vi "Read XML HW Configuration File.vi"(8 "error in (no error)":errorcluster, 10 "XML Configuration File Path":path=path "D:/1553 CD/HW Reference files/1553_HW_Reference_001.xml") -> (0 "error out":errorcluster, 3 "channels":T1[](array[typedef]))   [LabVIEW 2020, in "Ballard 1553 System Explorer.lvlib"]
uses:
  Ballard 1553 System Explorer.lvlib
  Ballard_Channel.ctl
  Ballard_BC.ctl
  Ballard_message.ctl
  Ballard_messageType.ctl
  Ballard_CWD1.ctl
  Ballard_CWD2.ctl
  Ballard_minorFrame.ctl
  Ballard_majorFrame.ctl
  Ballard_acyclicFrame.ctl
  Ballard_RT.ctl
  Ballard_RT subAddress.ctl
  Ballard_RT direction.ctl
  Ballard_RT rtMode.ctl
  Ballard_RT modeCode.ctl
  C:/Users/Administrator/Desktop/GIT/Ballard-MIL-STD-1553-Custom-Device/Source/System Explorer/SubVIs/Parse XML Ballard/1.2/BTIXML_SerDes.dll
  1.2/BTIXML_SerDes.dll
panel:
  out "name":string
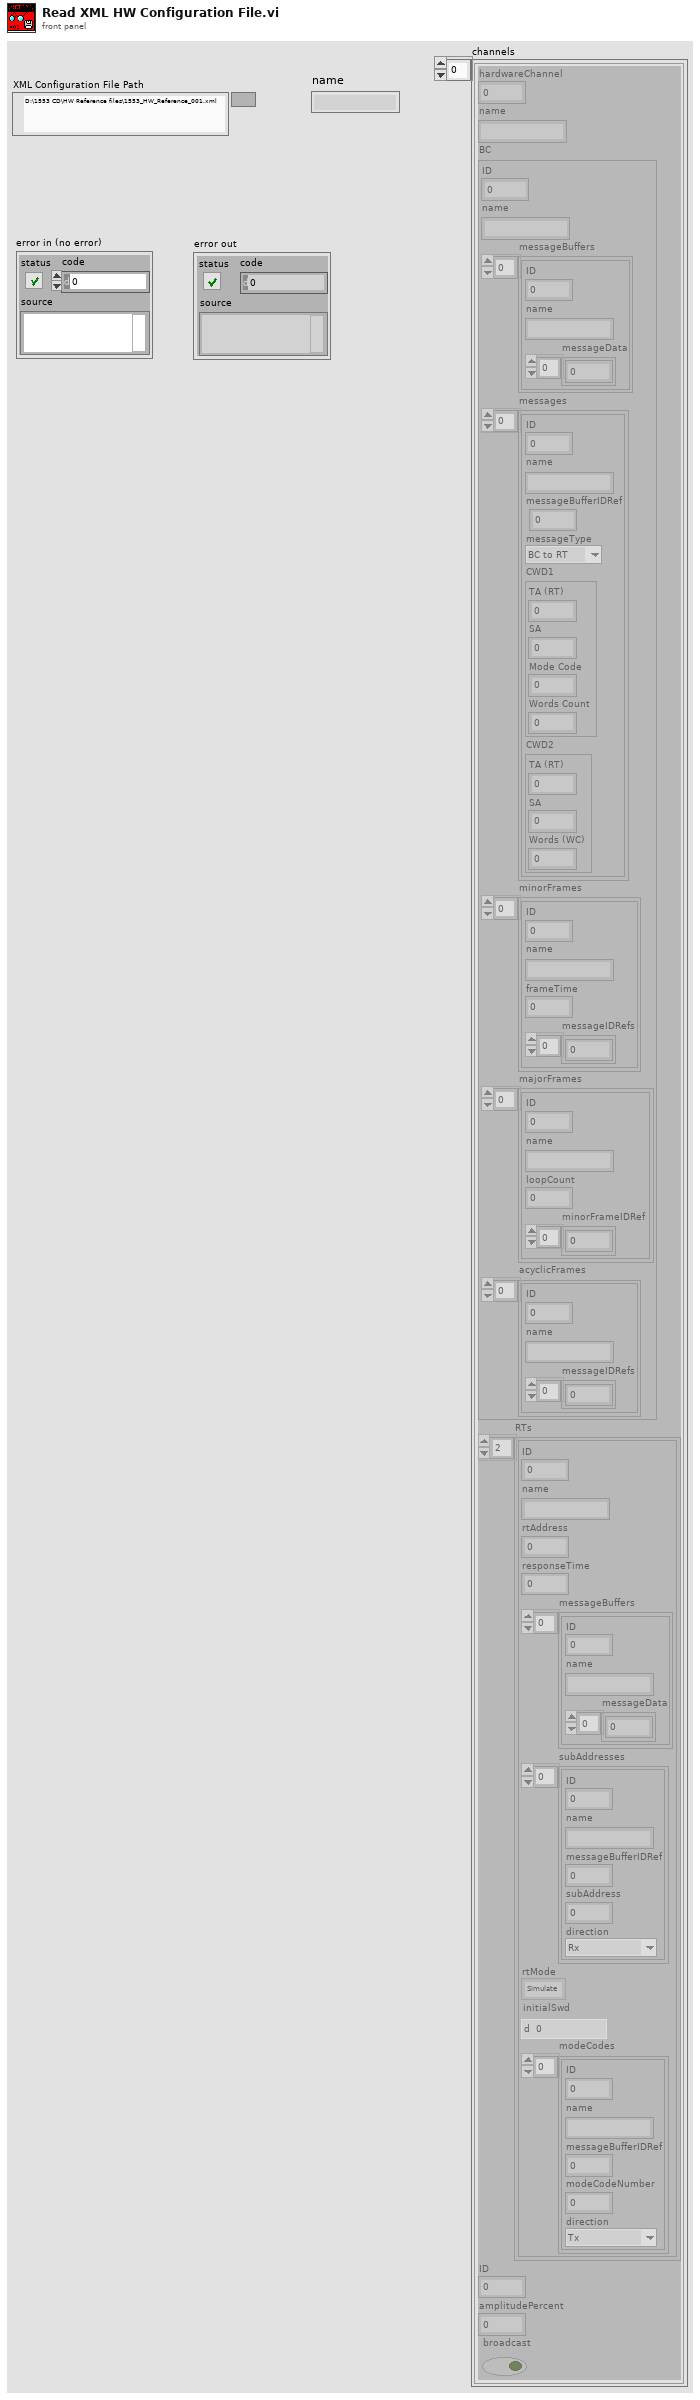
[diagram p1: front panel]
types:
  T1 = typedef "Ballard 1553 System Explorer.lvlib/Ballard_Channel.ctl" = cluster{"hardwareChannel":i32, "name":string, "BC":T2, "RTs":T10[], "ID":i32, "amplitudePercent":dbl, "broadcast":bool}
  T2 = typedef "Ballard 1553 System Explorer.lvlib/Ballard_BC.ctl" = cluster{"ID":i32, "name":string, "messageBuffers":cluster{"ID":i32, "name":string, "messageData":u16[]}[], "messages":T3[], "minorFrames":T7[], "majorFrames":T8[], "acyclicFrames":T9[]}
  T3 = typedef "Ballard 1553 System Explorer.lvlib/Ballard_message.ctl" = cluster{"ID":i32, "name":string, "messageBufferIDRef":i32, "messageType":T4, "CWD1":T5, "CWD2":T6}
  T4 = typedef "Ballard 1553 System Explorer.lvlib/Ballard_messageType.ctl" = enum16{"BC to RT", "RT to BC", "RT to RT", "MC (Rx)", "MC (Tx)"}
  T5 = typedef "Ballard 1553 System Explorer.lvlib/Ballard_CWD1.ctl" = cluster{"TA (RT)":i8, "SA":i8, "Mode Code":i8, "Words Count":i8}
  T6 = typedef "Ballard 1553 System Explorer.lvlib/Ballard_CWD2.ctl" = cluster{"TA (RT)":i8, "SA":i8, "Words (WC)":i8}
  T7 = typedef "Ballard 1553 System Explorer.lvlib/Ballard_minorFrame.ctl" = cluster{"ID":i32, "name":string, "frameTime":i32, "messageIDRefs":i32[]}
  T8 = typedef "Ballard 1553 System Explorer.lvlib/Ballard_majorFrame.ctl" = cluster{"ID":i32, "name":string, "loopCount":i32, "minorFrameIDRef":i32[]}
  T9 = typedef "Ballard 1553 System Explorer.lvlib/Ballard_acyclicFrame.ctl" = cluster{"ID":i32, "name":string, "messageIDRefs":i32[]}
  T10 = typedef "Ballard 1553 System Explorer.lvlib/Ballard_RT.ctl" = cluster{"ID":i32, "name":string, "rtAddress":i8, "responseTime":i32, "messageBuffers":cluster{"ID":i32, "name":string, "messageData":u16[]}[], "subAddresses":T11[], "rtMode":T13, "initialSwd":u16, "modeCodes":T14[]}
  T11 = typedef "Ballard 1553 System Explorer.lvlib/Ballard_RT subAddress.ctl" = cluster{"ID":i32, "name":string, "messageBufferIDRef":i32, "subAddress":i8, "direction":T12}
  T12 = typedef "Ballard 1553 System Explorer.lvlib/Ballard_RT direction.ctl" = enum16{"Tx", "Rx"}
  T13 = typedef "Ballard 1553 System Explorer.lvlib/Ballard_RT rtMode.ctl" = enum16{"Simulate", "Monitor", "Disable"}
  T14 = typedef "Ballard 1553 System Explorer.lvlib/Ballard_RT modeCode.ctl" = cluster{"ID":i32, "name":string, "messageBufferIDRef":i32, "modeCodeNumber":i8, "direction":T12}
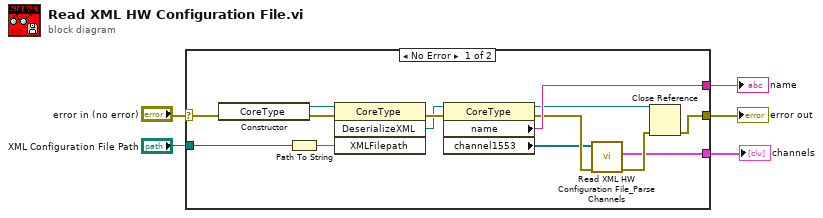
[diagram p0: block diagram]
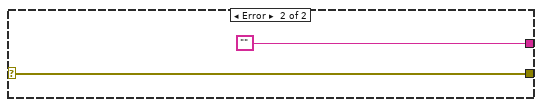
[diagram p2: hidden frame]
diagram:
  n1 = case shown="No Error" "error in (no error)" {
    selector: "error in (no error)" -> [w12 w21]
    tunnel: "XML Configuration File Path" -> [w19 _]
    tunnel: [w14 w21] -> w3
    tunnel: [w18 "" ("name")] -> w2
    tunnel: [w13 _] -> w1
    frame No Error {
      n2 = constructor class="CoreType"(error in=w12) -> (reference out=w6:refnum<k24>, error out=w7:errorcluster)  [unwired: 2 in, 1 out]
      n3 = Path To String(path=w19) -> (string=w10:string)
      n4 = invoke class="CoreType" method="DeserializeXML"(reference=w6, error in=w7, "XMLFilepath"=w10) -> (error out=w11:errorcluster, "DeserializeXML"=w9:refnum<k24>)  [unwired: 1 in, 2 out]
      n5 = property class="CoreType"(reference=w9, error in=w11) -> (reference out=w15:refnum<k24>, error out=w17:errorcluster, "name"=w18:string, "channel1553"=w8:refnum<k24>[])
      n6 = call "Read XML HW Configuration File_Parse Channels.vi"("error in (no error)"=w17, "channel1553"=w8) -> ("error out"=w16:errorcluster, "channels"=w13:T1[])  [unwired: 8 in]
      n7 = Close Reference(reference=w15, error in (no error)=w16) -> (error out=w14:errorcluster)
    }
    frame Error {
    }
  }
  "error out" <- w3
  "name" <- w2
  "channels" <- w1
